vi "Configure System.vi"   [LabVIEW 2014, in "Associated Power Technologies 8500 Series.lvlib"]
uses:
  <instrlib>/Associated Power Technologies 8500 Series/Associated Power Technologies 8500 Series.lvlib
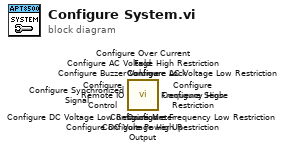
[diagram p0: block diagram]
diagram:
  n1 = call <instrlib>:"Configure Meter.vi"() -> ()  [unwired: 10 in, 2 out]
  n2 = call <instrlib>:"Configure Lock.vi"() -> ()  [unwired: 10 in, 2 out]
  n3 = call <instrlib>:"Configure Synchronized Signal.vi"() -> ()  [unwired: 10 in, 2 out]
  n4 = call <instrlib>:"Configure Sense.vi"() -> ()  [unwired: 10 in, 2 out]
  n5 = call <instrlib>:"Configure Power Up Output.vi"() -> ()  [unwired: 10 in, 2 out]
  n6 = call <instrlib>:"Configure Over Current Fold.vi"() -> ()  [unwired: 10 in, 2 out]
  n7 = call <instrlib>:"Configure Buzzer Volume.vi"() -> ()  [unwired: 10 in, 2 out]
  n8 = call <instrlib>:"Configure Frequency Low Restriction.vi"() -> ()  [unwired: 10 in, 2 out]
  n9 = call <instrlib>:"Configure Frequency High Restriction.vi"() -> ()  [unwired: 10 in, 2 out]
  n10 = call <instrlib>:"Configure DC Voltage Low Restriction.vi"() -> ()  [unwired: 10 in, 2 out]
  n11 = call <instrlib>:"Configure DC Voltage High Restriction.vi"() -> ()  [unwired: 10 in, 2 out]
  n12 = call <instrlib>:"Configure AC Voltage Low Restriction.vi"() -> ()  [unwired: 10 in, 2 out]
  n13 = call <instrlib>:"Configure AC Voltage High Restriction.vi"() -> ()  [unwired: 10 in, 2 out]
  n14 = call <instrlib>:"Configure Remote IO Control.vi"() -> ()  [unwired: 10 in, 2 out]
